vi "TTTRmain.vi"() -> ()   [LabVIEW 2011]
uses:
  Global.vi
  MT Scan/SubVIs/hhlib.dll
panel:
  out "Warnings":string
  out "Serial Num.":string
  in  "Ch4 Offs":i32 min=-99999 max=99999 step=1
  in  "Ch3 Offs":i32 min=-99999 max=99999 step=1
  in  "Ch2 Offs":i32 min=-99999 max=99999 step=1
  in  "Ch1 Offs":i32 min=-99999 max=99999 step=1
  in  "Sync Offs":i32 min=-99999 max=99999 step=1
  out "Rate 4":i32(slide) scale=0.01..100000000.0 scale format="%.0e"
  in  "Ch4 ZeroX":i32=10 min=0 max=20 step=1
  in  "Ch4 Level":i32=50 min=0 max=800 step=10
  out "Rate 3":i32(slide) scale=0.01..100000000.0 scale format="%.0e"
  in  "Ch3 ZeroX":i32=10 min=0 max=20 step=1
  in  "Ch3 Level":i32=50 min=0 max=800 step=10
  in  "Ch2 ZeroX":i32=10 min=0 max=20 step=1
  in  "Ch2 Level":i32=50 min=0 max=800 step=10
  out "Rate 2":i32(slide) scale=0.01..100000000.0 scale format="%.0e"
  out "DeviceIndex":i32=-1
  out "Rate 1":i32(slide) scale=0.01..100000000.0 scale format="%.0e"
  in  "Acq.Time":i32=10000 min=1 max=3600000 step=100
  in  "Binning":i32 min=0 max=10 step=1
  in  "Ch1 ZeroX":i32=10 min=0 max=20 step=1
  in  "Ch1 Level":i32=50 min=0 max=800 step=10
  in  "Sync ZeroX":i32=10 min=0 max=20 step=1
  in  "Sync Level":i32=50 min=0 max=800 step=10
  in  "Syncdiv":enum16{"1", "2", "4", "8"}(ring)
  out "file error status":errorcluster
  in  "File path":path=path "c:/test"
  out "FiFoOverrun":bool
  out "Progress":i32
  out "DLL Version (must be 1.2)":string caption="DLL Version"
  out "Sync Rate":i32(slide) scale=0.01..100000000.0 scale format="%.0e"
  out "Resolution":dbl min=0.0 max=2000.0 step=1.0 format="%.2f"
  out "Calibration Status":string
  in  "Run":bool
  out "Initialization Status":string
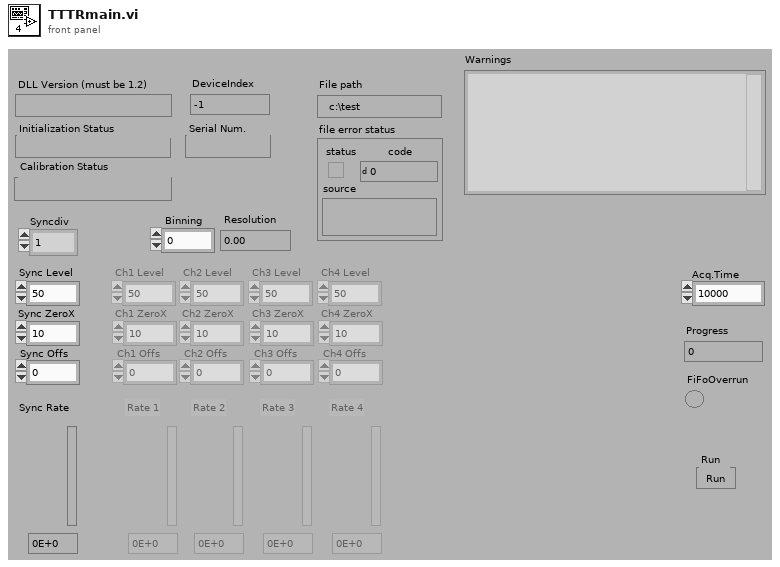
[diagram p1: front panel]
types:
  T1 = cluster{"rate":i32, "rate":i32, "rate":i32, "rate":i32, "rate":i32, "rate":i32, "rate":i32, "rate":i32}
  T2 = enum16{"open", "replace", "create", "open or create", "replace or create", "replace or create with confirmation"}
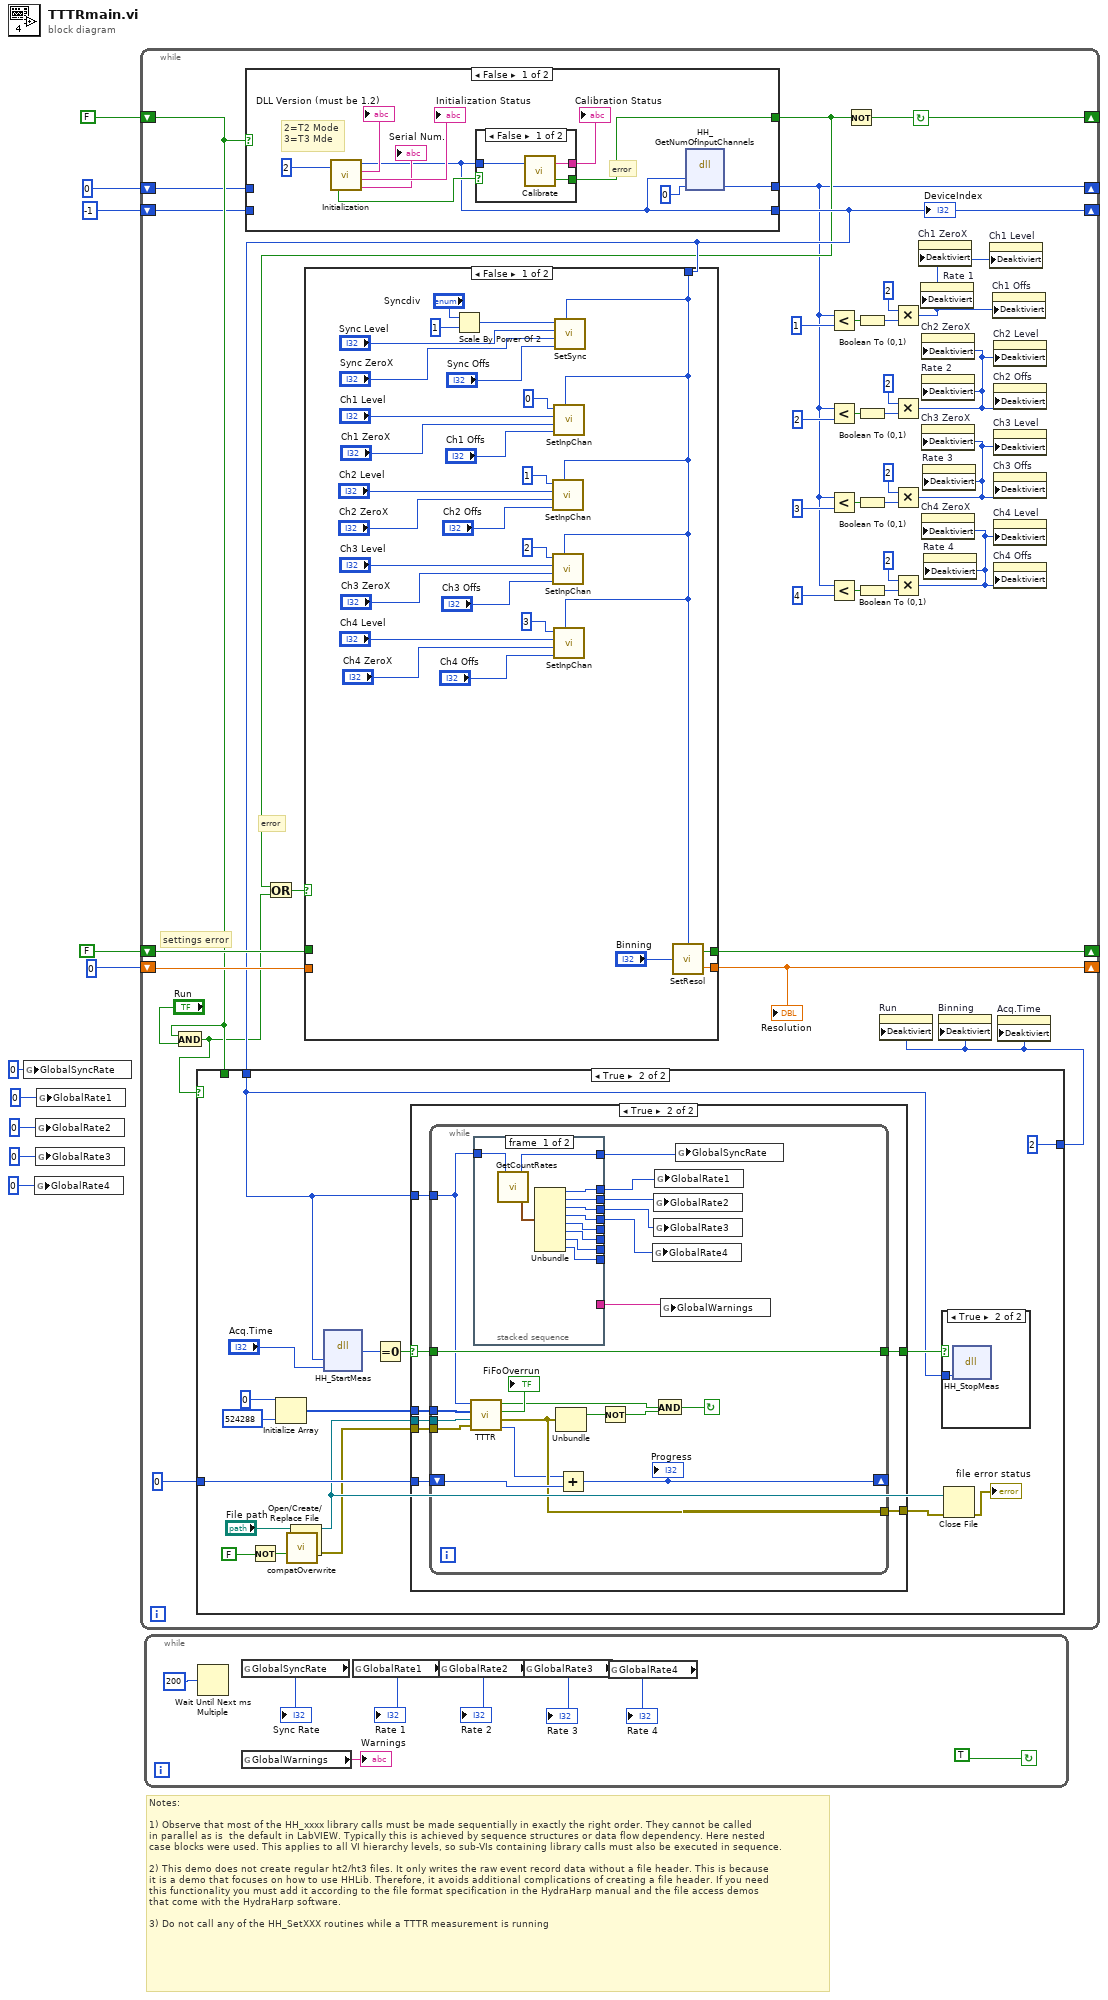
[diagram p0: block diagram]
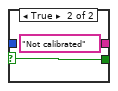
[diagram p2: hidden frame]
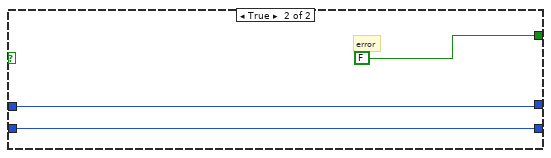
[diagram p3: hidden frame]
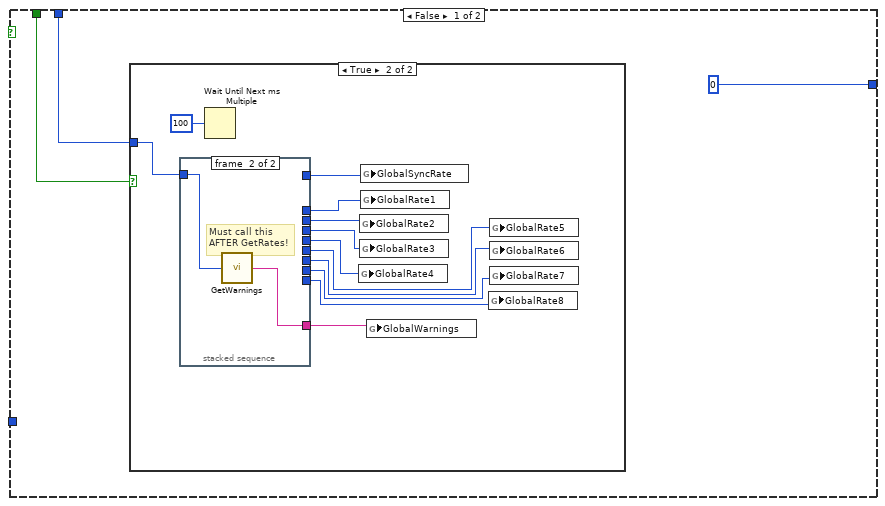
[diagram p4: hidden frame]
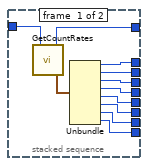
[diagram p6: hidden frame]
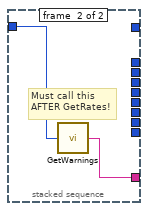
[diagram p8: hidden frame]
diagram:
  # "Notes: \n\n1) Observe that most of the HH_xxxx library calls must be made sequentially in exactly the right order. They cannot be called \nin parallel as is  the default in LabVIEW. Typically this is achieved by sequence structures or data flow dependency. Here nested \ncase blocks were used. This applies to all VI hierarchy levels, so sub-VIs containing library calls must also be executed in sequence.\n\n2) This demo does not create regular ht2/ht3 files. It only writes the raw event record data without a file header. This is because \nit is a demo that focuses on how to use HHLib. Therefore, it avoids additional complications of creating a file header. If you need \nthis functionality you must add it according to the file format specification in the HydraHarp manual and the file access demos \nthat come with the HydraHarp software. \n\n3) Do not call any of the HH_SetXXX routines while a TTTR measurement is running"
  n1 = global write "Global.vi" "GlobalSyncRate"(0) -> ()
  n2 = global write "Global.vi" "GlobalRate4"(0) -> ()
  n3 = global write "Global.vi" "GlobalRate2"(0) -> ()
  n4 = global write "Global.vi" "GlobalRate3"(0) -> ()
  n5 = global write "Global.vi" "GlobalRate1"(0) -> ()
  n6 = while {
    shift-left: 0 -> [w12]
    shift-right: [w11] -> _
    shift-left: -1 -> [w38]
    shift-right: [w37] -> _
    shift-left: FALSE -> [w40]
    shift-right: [w41] -> _
    shift-left: 0 -> [w44]
    shift-right: [w45] -> _
    shift-left: FALSE -> [w43]
    shift-right: [w46] -> _
    stop <- w41 continue-if-true
    # "settings error"
    # "error"
    n7 = And(x=w40, y="Run") -> (x .and. y?=w15:bool)
    n8 = case shown="False" w40 {
      tunnel: [w55 FALSE] -> w14
      tunnel: [w48 w63] -> w37
      tunnel: w38 -> [_ w63]
      tunnel: [w47 w62] -> w11
      tunnel: w12 -> [_ w62]
      frame False {
        # "2=T2 Mode\n3=T3 Mde"
        # "error"
        n9 = call "Initialization.vi"("Mode"=2) -> ("Initialisation Error"=w50:bool, "Deviceindex"=w48:i32, "DLL Version"=→"DLL Version (must be 1.2)":string, "Initialization Status"=→"Initialization Status":string, "Serial[8]"=→"Serial Num.":string)
        n10 = case shown="False" w50 {
          selector: w50 -> [_ w60]
          tunnel: [w59 "Not calibrated"] -> w56
          tunnel: [w58 w60] -> w55
          tunnel: w48 -> [w57 _]
          frame False {
            n11 = call "Calibrate.vi"("Deviceindex"=w57) -> ("Calib Error"=w58:bool, "Status"=w59:string)  [unwired: 1 in]
          }
          frame True {
          }
        }
        "Calibration Status" <- w56
        n12 = dll-call lib="C:/Users/Core-FCS/Desktop/AbelFCS/MT Scan/SubVIs/hhlib.dll" fn="HH_GetNumOfInputChannels" label="HH_GetNumOfCh"("devidx"=w48, "numch"=0) -> ("numch"=w47:i32)  [unwired: 5 in, 2 out]
      }
      frame True {
        # "error"
      }
    }
    "DeviceIndex" <- w37
    n13 = case shown="True" w15 {
      tunnel: 0 -> [_ w109]
      tunnel: [0 2] -> w32
      tunnel: w40 -> [w66 _]
      tunnel: w37 -> [w65 w94]
      frame False {
        n14 = case shown="True" w66 {
          tunnel: w65 -> [_ w68]
          frame False {
          }
          frame True {
            n15 = stacked-sequence {
              tunnel: w68 -> [w90 w91]
              tunnel: [w89 _] -> w78
              tunnel: [w87 _] -> w77
              tunnel: [w86 _] -> w76
              tunnel: [w85 _] -> w75
              tunnel: [w84 _] -> w74
              tunnel: [w83 _] -> w73
              tunnel: [w82 _] -> w72
              tunnel: [w81 _] -> w71
              tunnel: [w80 _] -> w70
              tunnel: [_ w92] -> w69
              frame #0 {
                n16 = call "GetCountRates.vi"("DeviceIndex"=w90) -> ("SyncRate"=w89:i32, "Count Rates"=w88:T1)
                n17 = Unbundle(w88) -> ("rate"=w87:i32, "rate"=w86:i32, "rate"=w85:i32, "rate"=w84:i32, "rate"=w83:i32, "rate"=w82:i32, "rate"=w81:i32, "rate"=w80:i32)
              }
              frame #1 {
                # "Must call this\nAFTER GetRates!"
                n18 = call "GetWarnings.vi"("Deviceindex"=w91) -> ("warningstext"=w92:string)
              }
            }
            n19 = Wait Until Next ms Multiple(millisecond multiple=100) -> ()  [unwired: 1 out]
            n20 = global write "Global.vi" "GlobalRate4"(w74) -> ()
            n21 = global write "Global.vi" "GlobalRate2"(w76) -> ()
            n22 = global write "Global.vi" "GlobalRate3"(w75) -> ()
            n23 = global write "Global.vi" "GlobalSyncRate"(w78) -> ()
            n24 = global write "Global.vi" "GlobalRate1"(w77) -> ()
            n25 = global write "Global.vi" "GlobalWarnings"(w69) -> ()
            n26 = global write "Global.vi" "GlobalRate8"(w70) -> ()
            n27 = global write "Global.vi" "GlobalRate5"(w73) -> ()
            n28 = global write "Global.vi" "GlobalRate6"(w72) -> ()
            n29 = global write "Global.vi" "GlobalRate7"(w71) -> ()
          }
        }
      }
      frame True {
        n30 = Not(x=FALSE) -> (.not. x?=w107:bool)
        n31 = Initialize Array(u8 0, 524288) -> (w99:u8[])
        n32 = call <vilib>:"compatOverwrite.vi"("overwrite (F)"=w107) -> ("overwrite?"=w93:T2)
        n33 = Open/Create/Replace File(file path (use dialog)="File path", operation (0:open)=w93) -> (refnum out=w106:refnum<file>, error out=w103:errorcluster)  [unwired: 4 in, 1 out]
        n34 = dll-call lib="C:/Users/Core-FCS/Desktop/AbelFCS/MT Scan/SubVIs/hhlib.dll" fn="HH_StartMeas"("devidx"=w94, "tacq"="Acq.Time") -> (w98:i32)  [unwired: 5 in, 2 out]
        n35 = Equal To 0?(x=w98) -> (x = 0?=w97:bool)
        n36 = case shown="True" w97 {
          selector: w97 -> [w112 w120]
          tunnel: [w112 w119] -> w110
          tunnel: w109 -> [_ w118]
          tunnel: w106 -> [_ w117]
          tunnel: w103 -> [w111 w116]
          tunnel: [w111 w115] -> w105
          tunnel: w99 -> [_ w114]
          tunnel: w94 -> [_ w113]
          frame False {
          }
          frame True {
            n37 = while {
              tunnel: w113 -> [w127]
              tunnel: w114 -> [w132]
              tunnel: [w136] -> w115
              tunnel: w116 -> [w130]
              tunnel: w117 -> [w131]
              shift-left: w118 -> [w139]
              shift-right: [w134] -> _
              tunnel: [w140] -> w119
              tunnel: w120 -> [w140]
              stop <- w129 continue-if-true
              n38 = call "TTTR.vi"("error in (no error)"=w130, "file refnum"=w131, "Array"=w132, "DeviceIndex"=w127) -> ("count"=w133:i32, "error out"=w136:errorcluster, "FiFoOverrun"=→"FiFoOverrun":bool, "OK"=w128:bool)
              n39 = stacked-sequence {
                tunnel: w127 -> [w151 w153]
                tunnel: [w150 _] -> w126
                tunnel: [w148 _] -> w125
                tunnel: [w147 _] -> w124
                tunnel: [w146 _] -> w123
                tunnel: [w145 _] -> w122
                tunnel: [w144 _] -> _
                tunnel: [w143 _] -> _
                tunnel: [w142 _] -> _
                tunnel: [w141 _] -> _
                tunnel: [_ w152] -> w121
                frame #0 {
                  n40 = call "GetCountRates.vi"("DeviceIndex"=w151) -> ("SyncRate"=w150:i32, "Count Rates"=w149:T1)
                  n41 = Unbundle(w149) -> ("rate"=w148:i32, "rate"=w147:i32, "rate"=w146:i32, "rate"=w145:i32, "rate"=w144:i32, "rate"=w143:i32, "rate"=w142:i32, "rate"=w141:i32)
                }
                frame #1 {
                  # "Must call this\nAFTER GetRates!"
                  n42 = call "GetWarnings.vi"("Deviceindex"=w153) -> ("warningstext"=w152:string)
                }
              }
              n43 = Unbundle(w136) -> ("status"=w135:bool)  [unwired: 2 out]
              n44 = Add(x=w133, y=w139) -> (x+y=w134:i32)
              "Progress" <- w134
              n45 = Not(x=w135) -> (.not. x?=w137:bool)
              n46 = global write "Global.vi" "GlobalRate4"(w122) -> ()
              n47 = global write "Global.vi" "GlobalRate2"(w124) -> ()
              n48 = global write "Global.vi" "GlobalRate3"(w123) -> ()
              n49 = global write "Global.vi" "GlobalRate1"(w125) -> ()
              n50 = And(x=w128, y=w137) -> (x .and. y?=w129:bool)
              n51 = global write "Global.vi" "GlobalWarnings"(w121) -> ()
              n52 = global write "Global.vi" "GlobalSyncRate"(w126) -> ()
            }
          }
        }
        n53 = case shown="True" w110 {
          tunnel: w94 -> [_ w154]
          frame False {
          }
          frame True {
            n54 = dll-call lib="C:/Users/Core-FCS/Desktop/AbelFCS/MT Scan/SubVIs/hhlib.dll" fn="HH_StopMeas"("devidx"=w154) -> ()  [unwired: 5 in, 2 out]
          }
        }
        n55 = Close File(refnum=w106, error in=w105) -> (error out=→"file error status":errorcluster)  [unwired: 1 out]
      }
    }
    n56 = Or(x=w14, y=w15) -> (x .or. y?=w13:bool)
    n57 = case shown="False" w13 {
      tunnel: [w161 w182] -> w46
      tunnel: w43 -> [_ w182]
      tunnel: [w160 w181] -> w45
      tunnel: w44 -> [_ w181]
      tunnel: w37 -> [w155 _]
      frame False {
        n58 = Scale By Power Of 2(n="Syncdiv", x=1) -> (x*2^n=w178:i32)
        n59 = call "SetInpChan.vi"("Channel"=1, "CFD Level"="Ch2 Level", "CFD ZeroX"="Ch2 ZeroX", "Offset"="Ch2 Offs", "DeviceIndex"=w155) -> ()  [unwired: 1 in, 1 out]
        n60 = call "SetInpChan.vi"("Channel"=2, "CFD Level"="Ch3 Level", "CFD ZeroX"="Ch3 ZeroX", "Offset"="Ch3 Offs", "DeviceIndex"=w155) -> ()  [unwired: 1 in, 1 out]
        n61 = call "SetInpChan.vi"("Channel"=0, "CFD Level"="Ch1 Level", "CFD ZeroX"="Ch1 ZeroX", "Offset"="Ch1 Offs", "DeviceIndex"=w155) -> ()  [unwired: 1 in, 1 out]
        n62 = call "SetInpChan.vi"("Channel"=3, "CFD Level"="Ch4 Level", "CFD ZeroX"="Ch4 ZeroX", "Offset"="Ch4 Offs", "DeviceIndex"=w155) -> ()  [unwired: 1 in, 1 out]
        n63 = call "SetSync.vi"("SyncDiv"=w178, "CFD Level"="Sync Level", "CFD ZeroX"="Sync ZeroX", "Offset"="Sync Offs", "DeviceIndex"=w155) -> ()  [unwired: 1 in, 1 out]
        n64 = call "SetResol.vi"("DeviceIndex"=w155, "Binning"="Binning") -> ("Resolution"=w160:dbl, "Error"=w161:bool)  [unwired: 2 in]
      }
      frame True {
      }
    }
    "Resolution" <- w45
    n65 = Less?(x=w11, y=1) -> (x < y?=w35:bool)
    n66 = Less?(x=w11, y=2) -> (x < y?=w29:bool)
    n67 = Less?(x=w11, y=3) -> (x < y?=w25:bool)
    n68 = Less?(x=w11, y=4) -> (x < y?=w21:bool)
    n69 = Not(x=w14) -> (.not. x?=w41:bool)
    n70 = Boolean To (0,1)(Boolean=w35) -> (0, 1=w34:i16)
    n71 = Boolean To (0,1)(Boolean=w29) -> (0, 1=w30:i16)
    n72 = Boolean To (0,1)(Boolean=w25) -> (0, 1=w26:i16)
    n73 = Boolean To (0,1)(Boolean=w21) -> (0, 1=w22:i16)
    n74 = property on="Run" class="Bool"("Deaktiviert"=w32) -> ()  [unwired: 2 in, 2 out]
    n75 = Multiply(x=2, y=w34) -> (x*y=w16:i32)
    n76 = Multiply(x=2, y=w30) -> (x*y=w17:i32)
    n77 = Multiply(x=2, y=w26) -> (x*y=w18:i32)
    n78 = Multiply(x=2, y=w22) -> (x*y=w19:i32)
    n79 = property on="Ch1 ZeroX" class="DigNum (strict)"("Deaktiviert"=w16) -> ()  [unwired: 2 in, 2 out]
    n80 = property on="Rate 1" class="Slide (strict)"("Deaktiviert"=w16) -> ()  [unwired: 2 in, 2 out]
    n81 = property on="Ch2 ZeroX" class="DigNum (strict)"("Deaktiviert"=w17) -> ()  [unwired: 2 in, 2 out]
    n82 = property on="Rate 2" class="Slide (strict)"("Deaktiviert"=w17) -> ()  [unwired: 2 in, 2 out]
    n83 = property on="Ch3 ZeroX" class="DigNum (strict)"("Deaktiviert"=w18) -> ()  [unwired: 2 in, 2 out]
    n84 = property on="Ch4 ZeroX" class="DigNum (strict)"("Deaktiviert"=w19) -> ()  [unwired: 2 in, 2 out]
    n85 = property on="Rate 3" class="Slide (strict)"("Deaktiviert"=w18) -> ()  [unwired: 2 in, 2 out]
    n86 = property on="Rate 4" class="Slide (strict)"("Deaktiviert"=w19) -> ()  [unwired: 2 in, 2 out]
    n87 = property on="Binning" class="DigNum (strict)"("Deaktiviert"=w32) -> ()  [unwired: 2 in, 2 out]
    n88 = property on="Ch1 Level" class="DigNum (strict)"("Deaktiviert"=w16) -> ()  [unwired: 2 in, 2 out]
    n89 = property on="Ch1 Offs" class="DigNum (strict)"("Deaktiviert"=w16) -> ()  [unwired: 2 in, 2 out]
    n90 = property on="Ch2 Level" class="DigNum (strict)"("Deaktiviert"=w17) -> ()  [unwired: 2 in, 2 out]
    n91 = property on="Ch2 Offs" class="DigNum (strict)"("Deaktiviert"=w17) -> ()  [unwired: 2 in, 2 out]
    n92 = property on="Ch3 Level" class="DigNum (strict)"("Deaktiviert"=w18) -> ()  [unwired: 2 in, 2 out]
    n93 = property on="Ch3 Offs" class="DigNum (strict)"("Deaktiviert"=w18) -> ()  [unwired: 2 in, 2 out]
    n94 = property on="Ch4 Level" class="DigNum (strict)"("Deaktiviert"=w19) -> ()  [unwired: 2 in, 2 out]
    n95 = property on="Ch4 Offs" class="DigNum (strict)"("Deaktiviert"=w19) -> ()  [unwired: 2 in, 2 out]
    n96 = property on="Acq.Time" class="DigNum (strict)"("Deaktiviert"=w32) -> ()  [unwired: 2 in, 2 out]
  }
  n97 = while {
    stop <- TRUE continue-if-true
    n98 = Wait Until Next ms Multiple(millisecond multiple=200) -> ()  [unwired: 1 out]
    n99 = global read "Global.vi" "GlobalSyncRate"() -> (→"Sync Rate":i32)
    n100 = global read "Global.vi" "GlobalWarnings"() -> (→"Warnings":string)
    n101 = global read "Global.vi" "GlobalRate1"() -> (→"Rate 1":i32)
    n102 = global read "Global.vi" "GlobalRate2"() -> (→"Rate 2":i32)
    n103 = global read "Global.vi" "GlobalRate3"() -> (→"Rate 3":i32)
    n104 = global read "Global.vi" "GlobalRate4"() -> (→"Rate 4":i32)
  }
